vi "Example Callback - Voltage Callback.vi"(4 "Voltage":refnum<user-event>, 5 "Event Data":T1, 6 "Control Ref":refnum<k24>, 7 "Event Common Data":T2) -> ()   [LabVIEW 2010]
uses:
  C:/tf/play/labview/Tinkerforge.dll
  Tinkerforge.dll
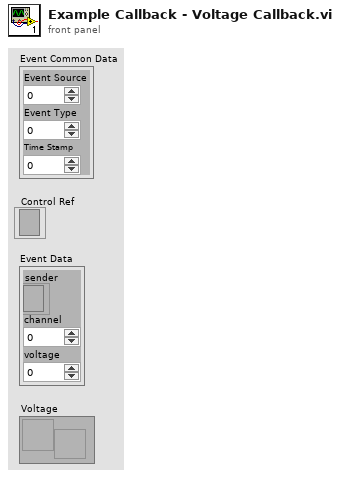
[diagram p1: front panel]
types:
  T1 = cluster{"sender":refnum<k24>, "channel":u8, "voltage":i32}
  T2 = cluster{"Event Source":i32, "Event Type":u32, "Time Stamp":u32}
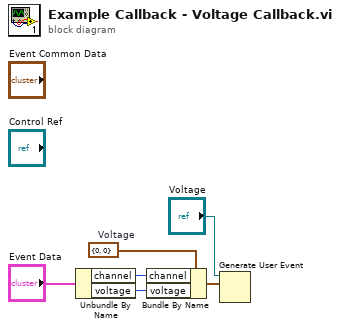
[diagram p0: block diagram]
diagram:
  w6 = cluster{"channel":u8, "voltage":i32} {"channel"=0, "voltage"=0}  # Voltage
  n1 = Unbundle By Name("Event Data") -> ("channel"=w4:u8, "voltage"=w3:i32)
  n2 = Bundle By Name(cluster=w6, "channel"=w4, "voltage"=w3) -> (w2:cluster{"channel":u8, "voltage":i32})
  n3 = Generate User Event(user event="Voltage", event data cluster=w2) -> ()  [unwired: 1 in, 2 out]
